vi "test.boolean_conversion.vi"   [LabVIEW 2020]
uses:
  <vilib>/addons/_JKI Toolkits/Caraya/classes/Assert/Assert Equal Value and Type_Variant.vi
  <vilib>/addons/_JKI Toolkits/Caraya/classes/Assert/Assert Equal Value_Variant.vi
  configuration-data/configuration-data.lvclass
  <vilib>/addons/_JKI Toolkits/Caraya/classes/Test/Test.lvclass
  <vilib>/addons/_JKI Toolkits/Caraya/classes/Assert/Assert.lvclass
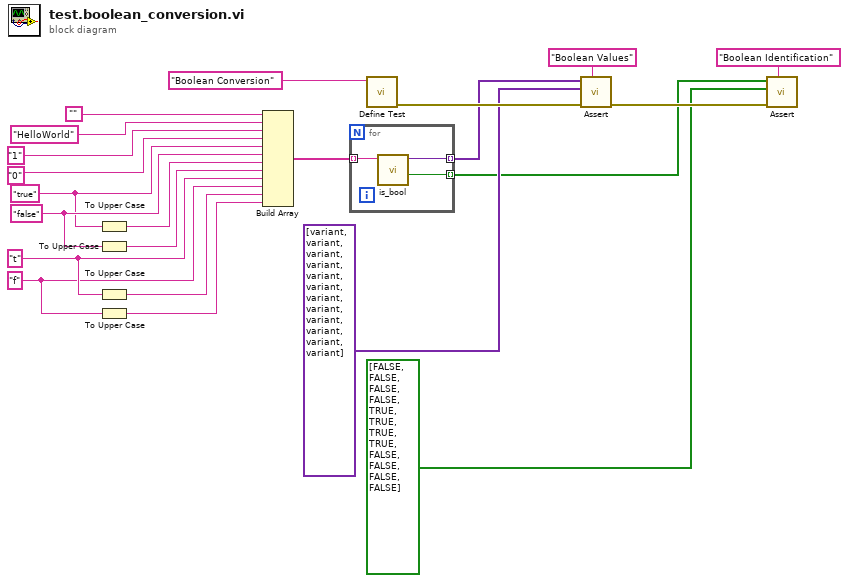
[diagram p0: block diagram]
diagram:
  w13 = "f"
  w15 = "t"
  w18 = "false"
  w11 = "true"
  n1 = To Upper Case(1:w11) -> (0:w17:string)
  n2 = To Upper Case(1:w18) -> (0:w16:string)
  n3 = To Upper Case(1:w15) -> (0:w14:string)
  n4 = To Upper Case(1:w13) -> (0:w12:string)
  n5 = Build Array("", "HelloWorld", "1", "0", w11, w18, w17, w16, w15, w13, w14, w12) -> (w10:string[])
  n6 = for {
    tunnel: w10 -> [w25] mode=indexing
    tunnel: [w24] -> w2 mode=indexing
    tunnel: [w23] -> w4 mode=indexing
    n7 = call "is_bool.vi"("data in"=w25) -> ("confirmed?"=w24:bool, "data out"=w23:variant)  [unwired: 9 in]
  }
  n8 = call <vilib>:"Define Test.vi"("Label (VI Title)"="Boolean Conversion") -> ("error out"=w7:errorcluster)  [unwired: 10 in]
  n9 = call-poly <vilib>:"Assert.vi"("Label"="Boolean Values", "error in (no error)"=w7, "Y"=variant[] [variant, variant, variant, variant, variant(bool TRUE), variant(bool FALSE), variant(bool TRUE), variant(bool FALSE), variant, variant, variant, variant] ("Array"), "X"=w4) -> ("error out"=w5:errorcluster)  [unwired: 7 in]
  n10 = call-poly <vilib>:"Assert.vi"("Label"="Boolean Identification", "error in (no error)"=w5, "Y"=bool[] [FALSE, FALSE, FALSE, FALSE, TRUE, TRUE, TRUE, TRUE, FALSE, FALSE, FALSE, FALSE] ("Array"), "X"=w2) -> ()  [unwired: 7 in, 1 out]
